vi "Field Drawing.vi"() -> (2 "2D Picture":picture)   [LabVIEW 2013]
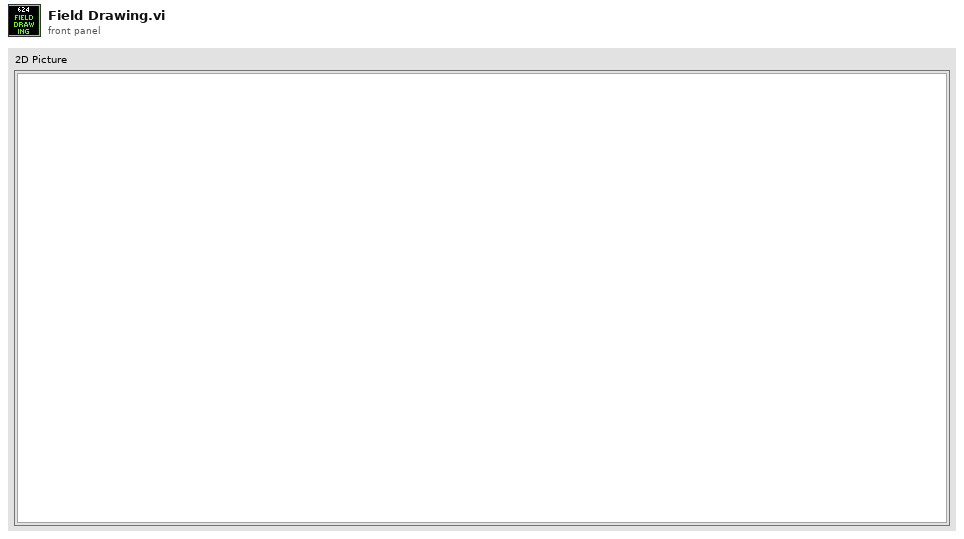
[diagram p1: front panel]
types:
  T1 = cluster{"left":i16, "top":i16, "right":i16, "bottom":i16}
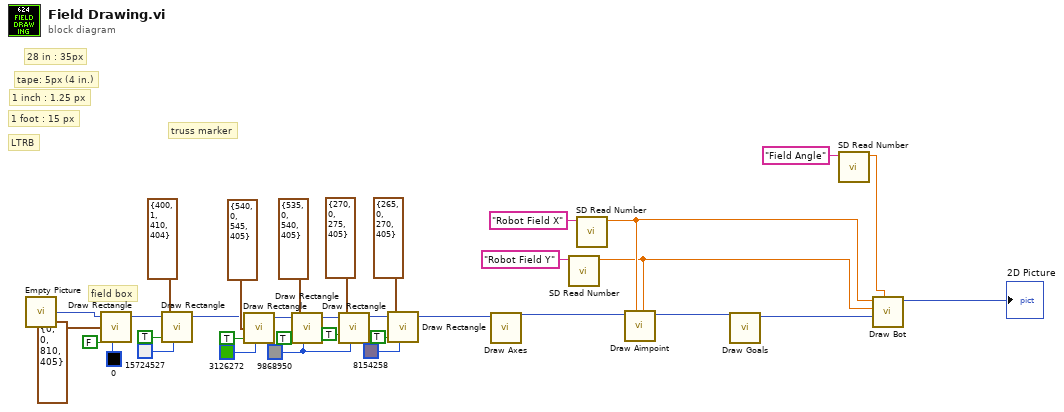
[diagram p0: block diagram]
diagram:
  w18 = u32 9868950 ("color(black)")
  # "28 in : 35px"
  # "tape: 5px (4 in.)"
  # "1 inch : 1.25 px"
  # "1 foot : 15 px"
  # "truss marker"
  # "LTRB"
  # "field box"
  n1 = call "Empty Picture"() -> ("empty picture"=w34:picture)
  n2 = call <vilib>:"Draw Rectangle.vi"("picture"=w34, "rect"=T1 {"left"=0, "top"=0, "right"=810, "bottom"=405}, "fill?(F)"=FALSE, "color(black)"=u32 0) -> ("new picture"=w30:picture)  [unwired: 5 in]
  n3 = call <vilib>:"Draw Rectangle.vi"("picture"=w30, "rect"=T1 {"left"=400, "top"=1, "right"=410, "bottom"=404}, "fill?(F)"=TRUE, "color(black)"=u32 15724527) -> ("new picture"=w26:picture)  [unwired: 5 in]
  n4 = call <vilib>:"Draw Rectangle.vi"("picture"=w26, "rect"=T1 {"left"=540, "top"=0, "right"=545, "bottom"=405}, "fill?(F)"=TRUE, "color(black)"=u32 3126272) -> ("new picture"=w23:picture)  [unwired: 5 in]
  n5 = call <vilib>:"Draw Rectangle.vi"("picture"=w23, "rect"=T1 {"left"=535, "top"=0, "right"=540, "bottom"=405}, "fill?(F)"=TRUE, "color(black)"=w18) -> ("new picture"=w20:picture)  [unwired: 5 in]
  n6 = call <vilib>:"Draw Rectangle.vi"("picture"=w20, "rect"=T1 {"left"=270, "top"=0, "right"=275, "bottom"=405}, "fill?(F)"=TRUE, "color(black)"=w18) -> ("new picture"=w16:picture)  [unwired: 5 in]
  n7 = call <vilib>:"Draw Rectangle.vi"("picture"=w16, "rect"=T1 {"left"=265, "top"=0, "right"=270, "bottom"=405}, "fill?(F)"=TRUE, "color(black)"=u32 8154258) -> ("new picture"=w10:picture)  [unwired: 5 in]
  n8 = call "Draw Axes.vi"("new picture in"=w10) -> ("new picture out"=w3:picture)  [unwired: 10 in]
  n9 = call <vilib>:"SD Read Number.vi"("Name"="Robot Field Y") -> ("Numeric"=w1:dbl)  [unwired: 8 in, 2 out]
  n10 = call <vilib>:"SD Read Number.vi"("Name"="Robot Field X") -> ("Numeric"=w2:dbl)  [unwired: 8 in, 2 out]
  n11 = call "Draw Aimpoint.vi"("Robot Y"=w1, "Robot X"=w2, "new picture in"=w3) -> ("out"=w4:picture)  [unwired: 8 in]
  n12 = call "Draw Goals.vi"("2D Picture"=w4) -> ("2D Picture 2"=w5:picture)  [unwired: 10 in]
  n13 = call <vilib>:"SD Read Number.vi"("Name"="Field Angle") -> ("Numeric"=w8:dbl)  [unwired: 8 in, 2 out]
  n14 = call "Draw Bot.vi"("Angle"=w8, "new picture in"=w5, "Robot Y"=w1, "Robot X"=w2) -> ("new picture out"=→"2D Picture":picture)  [unwired: 7 in]
